vi "Initialize Global Analog.vi"(0 "System no.":i32=1 min=1 step=1, 5 "error in":errorcluster) -> (19 "error out":errorcluster)   [LabVIEW 2020]
doc: "This VI initializes Global Analog according to the given system no. \n\nValid for Analog systems."
uses:
  Global Analog.vi
panel:
  # "This vi initializes Global Analog\naccording to the given system no."
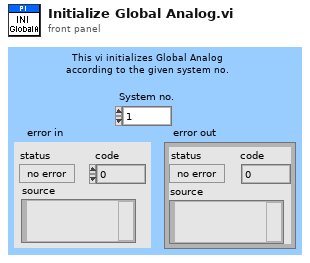
[diagram p1: front panel]
types:
  T1 = cluster{"Conversion factor":dbl[], "Velocity":dbl[], "Velocity control mode":bool, "AO.Resolution":dbl, "Lower voltage limit (V)":dbl, "Upper voltage limit (V)":dbl, "AO_WF_T (s)":dbl, "AI Sample Rate":dbl, "AI Samples/Channel":i32, "Hyperbit":bool, "Offset (V)":dbl[], "Hyperbit StayOnPos":bool, "Gain (V)":dbl[], "Bit rate (Hz)":dbl, "PWM rate (Hz)":dbl, "HyperBit Password":string, "AO.MaxRate":dbl, "Conversion offset":dbl[]}[]
  T2 = cluster{"Conversion factor":dbl[], "Velocity":dbl[], "Velocity control mode":bool, "AO.Resolution":dbl, "Lower voltage limit (V)":dbl, "Upper voltage limit (V)":dbl, "AO_WF_T (s)":dbl, "AI Sample Rate":dbl, "AI Samples/Channel":i32, "Hyperbit":bool, "Offset (V)":dbl[], "Hyperbit StayOnPos":bool, "Gain (V)":dbl[], "Bit rate (Hz)":dbl, "PWM rate (Hz)":dbl, "HyperBit Password":string, "AO.MaxRate":dbl, "Conversion offset":dbl[]}
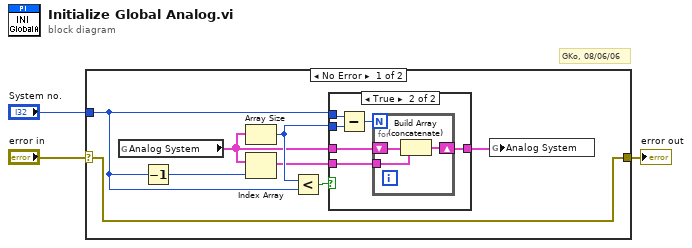
[diagram p0: block diagram]
diagram:
  # "GKo, 08/06/06"
  n1 = case shown="No Error" "error in" {
    selector: "error in" -> [w4 w22]
    tunnel: "System no." -> [w10 _]
    tunnel: [w4 w22] -> w1
    frame No Error {
      n2 = global read "Global Analog.vi" "Analog System"() -> (w6:T1)
      n3 = Decrement(x=w10) -> (x-1=w8:i32)
      n4 = Array Size(array=w6) -> (size(s)=w9:i32)
      n5 = Index Array(array=w6, index=w8) -> (element=w7:T2)
      n6 = Less?(x=w9, y=w10) -> (x < y?=w11:bool)
      n7 = case shown="True" w11 {
        tunnel: w10 -> [_ w17]
        tunnel: w9 -> [_ w16]
        tunnel: w6 -> [w12 w15]
        tunnel: w7 -> [_ w14]
        tunnel: [w12 w13] -> w5
        frame False {
        }
        frame True {
          n8 = Subtract(x=w17, y=w16) -> (x-y=w18:i32)
          n9 = for {
            N: w18 -> [_]
            shift-right: [w21] -> w13
            shift-left: w15 -> [w20]
            tunnel: w14 -> [w19]
            n10 = Build Array (concatenate)(w20, w19) -> (w21:T1)
          }
        }
      }
      n11 = global write "Global Analog.vi" "Analog System"(w5) -> ()
    }
    frame Error {
    }
  }
  "error out" <- w1
